vi "util.proc.init.vi"(8 "error in":errorcluster, 10 "Proc Path":path, 11 "Procedure in":variant[](array[variant])) -> (0 "error out":errorcluster, 3 "Procedure out":variant[](array[variant]))   [LabVIEW 2024]
uses:
  controls/typeProcVarientName.ctl
  Polymorphics/variantCtrlString.vi
  <vilib>/Utility/error.llb/Clear Errors.vi
  <vilib>/Utility/error.llb/Trim Whitespace.vi
  proc.util.validateParamExist.vi
  <vilib>/Utility/error.llb/Trim Whitespace One-Sided.vi
  <vilib>/Utility/libraryn.llb/Create Directory Recursive.vi
  util.error.create.vi
panel:
  out "Module Name":string
  out "result string":string
  out "before substring":string
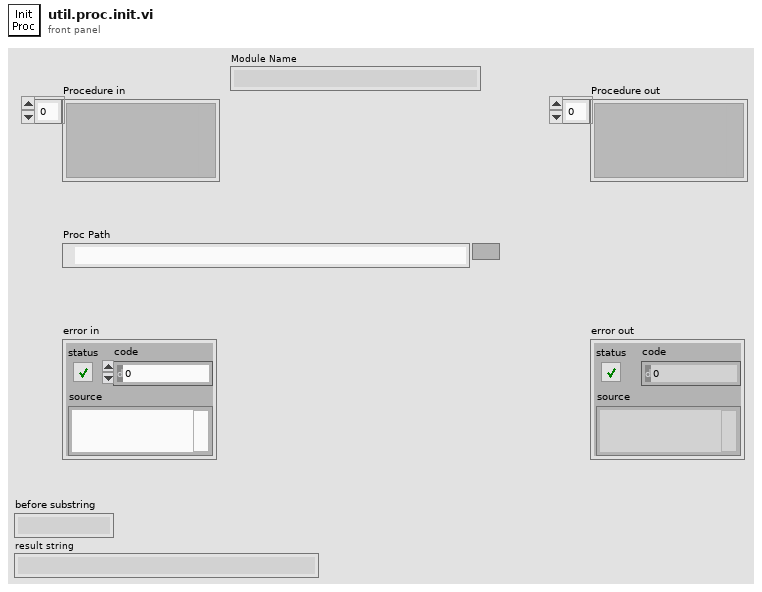
[diagram p1: front panel]
types:
  T1 = typedef "typeProcVarientName.ctl" = enum16{"procNameID", "procModuleID", "procPath", "procIsRunning", "procIndex", "procModule", "procRegisterNumeric", "procRegisterString", "procReport", "procReportPrev", "procCLK", "procStepPointer", "procType"}
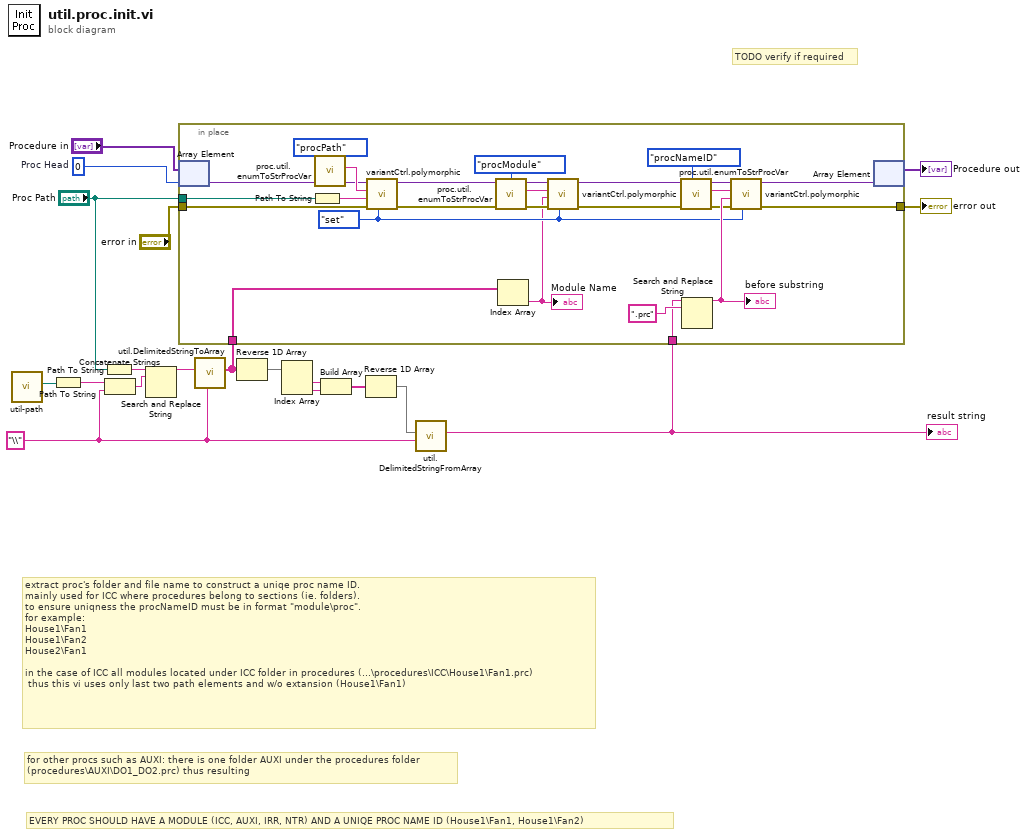
[diagram p0: block diagram]
diagram:
  w5 = "\\" ("string")
  w17 = 0  # Proc Head
  # "EVERY PROC SHOULD HAVE A MODULE (ICC, AUXI, IRR, NTR) AND A UNIQE PROC NAME ID (House1\\Fan1, House1\\Fan2)"
  # "for other procs such as AUXI: there is one folder AUXI under the procedures folder\n(procedures\\AUXI\\DO1_DO2.prc) thus resulting"
  # "extract proc's folder and file name to construct a uniqe proc name ID.\nmainly used for ICC where procedures belong to sections (ie. folders).\nto ensure uniqness the procNameID must be in format \"module\\proc\".\nfor example:\nHouse1\\Fan1\nHouse1\\Fan2\nHouse2\\Fan1\n\nin the case of ICC all modules located under ICC folder in procedures (...\\procedures\\ICC\\House1\\Fan1.prc) \n thus this vi uses only last two path elements and w/o extansion (House1\\Fan1)"
  # "TODO verify if required"
  n1 = call "util-path.vi"() -> ("SelectedPath"=w12:path)  [unwired: 7 in, 4 out]
  n2 = Path To String(path=w12) -> (string=w11:string)
  n3 = Path To String(path="Proc Path") -> (string=w13:string)
  n4 = Concatenate Strings(w11, w5) -> (w10:string)
  n5 = Search and Replace String(input string=w13, search string=w10) -> (result string=w2:string)  [unwired: 6 in, 3 out]
  n6 = call "util.DelimitedStringToArray.vi"("delimiter (,)"=w5, "delimitaed string"=w2) -> ("array out"=w1:string[])  [unwired: 9 in]
  n7 = Reverse 1D Array(array=w1) -> (reversed array=w9:string[])
  n8 = Index Array(array=w9) -> (element #1=w8:string, element #2=w7:string)  [unwired: 2 in]
  n9 = Build Array(w8, w7) -> (w6:string[])
  n10 = Reverse 1D Array(array=w6) -> (reversed array=w4:string[])
  n11 = call "util.DelimitedStringFromArray.vi"("delimiter (Comma)"=w5, "params array in"=w4) -> ("delimited string out"=w3:string)  [unwired: 9 in]
  "result string" <- w3
  n12 = in-place {
    in-place-border: "error in" -> [w38]
    in-place-border: [w34] -> w18
    in-place-border: "Proc Path" -> [w30]
    in-place-border: w3 -> [w29]
    in-place-border: w1 -> [w21]
    w22 = enum16{"get", "set"}."set" ("menu in (get)")
    n13 = in-place-array #1("Procedure in", w17) -> (w39:variant)
    n14 = Path To String(path=w30) -> (string=w37:string)
    n15 = call "proc.util.enumToStrProcVar.vi"("Proc var"=typeProcVarientName."procPath") -> ("String"=w41:string)  [unwired: 10 in]
    n16 = call-poly "variantCtrl.polymorphic.vi"("menu in (get)"=w22, "error in"=w38, "String Value"=w37, "name in"=w41, "Step in"=w39) -> ("error out"=w25:errorcluster, "Step out"=w27:variant)  [unwired: 3 in, 2 out]
    n17 = call "proc.util.enumToStrProcVar.vi"("Proc var"=typeProcVarientName."procModule") -> ("String"=w28:string)  [unwired: 10 in]
    n18 = Index Array(array=w21) -> (element=w20:string)  [unwired: 1 in]
    "Module Name" <- w20
    n19 = call-poly "variantCtrl.polymorphic.vi"("menu in (get)"=w22, "error in"=w25, "String Value"=w20, "name in"=w28, "Step in"=w27) -> ("error out"=w24:errorcluster, "Step out"=w26:variant)  [unwired: 3 in, 2 out]
    n20 = call "proc.util.enumToStrProcVar.vi"("Proc var"=typeProcVarientName."procNameID") -> ("String"=w35:string)  [unwired: 10 in]
    n21 = Search and Replace String(input string=w29, search string=".prc" ("regular expression")) -> (result string=w32:string)  [unwired: 6 in, 3 out]
    "before substring" <- w32
    n22 = call-poly "variantCtrl.polymorphic.vi"("menu in (get)"=w22, "error in"=w24, "String Value"=w32, "name in"=w35, "Step in"=w26) -> ("error out"=w34:errorcluster, "Step out"=w33:variant)  [unwired: 3 in, 2 out]
    n23 = in-place-array #1(w33) -> (→"Procedure out":variant[])  [unwired: 1 out]
  }
  "error out" <- w18
